vi "Read Sample DBL.vi"(11 "Virtual Sensor from CSV in":refnum<class "Virtual Sensor from CSV.lvclass">) -> (1 "Time Stamp":timestamp format="%<%x %.3X>T", 2 "Sample DBL":dbl, 3 "Virtual Sensor from CSV out":refnum<class "Virtual Sensor from CSV.lvclass">)   [LabVIEW 2024, in "Virtual Sensor from CSV.lvclass"]
uses:
  Virtual Sensor from CSV.lvclass
  Virtual Sensor from CSV.lvclass/Virtual Sensor from CSV.ctl
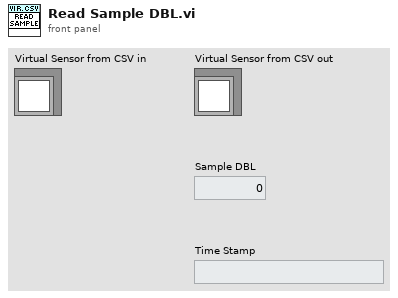
[diagram p1: front panel]
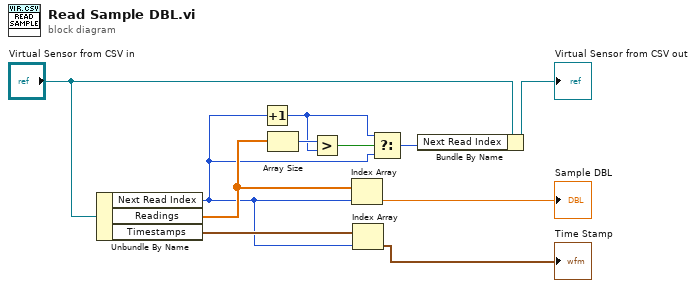
[diagram p0: block diagram]
diagram:
  n1 = Unbundle By Name("Virtual Sensor from CSV in") -> ("Next Read Index"=w7:i32, "Readings"=w10:dbl[], "Timestamps"=w11:timestamp[])
  n2 = Increment(x=w7) -> (x+1=w6:i32)
  n3 = Array Size(array=w10) -> (size(s)=w9:i32)
  n4 = Greater?(x=w9, y=w6) -> (0:w8:bool)
  n5 = Index Array(array=w10, index=w7) -> (element=→"Sample DBL":dbl)
  n6 = Index Array(array=w11, index=w7) -> (element=→"Time Stamp":timestamp)
  n7 = Select(t=w6, s=w8, f=w7) -> (s? t:f=w5:i32)
  n8 = Bundle By Name(cluster="Virtual Sensor from CSV in", "Next Read Index"=w5) -> (→"Virtual Sensor from CSV out":refnum<class "Virtual Sensor from CSV.lvclass">)
